vi "RW Limits Array.vi"(0 "Refnum In":T1, 2 "Read (F)":bool, 7 "LimitsArray In":cluster{"Step":dbl, "Max":dbl, "Min":dbl}[](array[cluster]), 11 "Error In":errorcluster) -> (4 "Refnum Out":T1, 8 "LimitsArray Out":cluster{"Step":dbl, "Max":dbl, "Min":dbl}[](array[cluster]), 15 "Error Out":errorcluster)   [LabVIEW 2013]
uses:
  <vilib>/Utility/config.llb/Config Data RefNum.ctl
  <vilib>/Utility/config.llb/Write Key (Double).vi
  <vilib>/Utility/config.llb/Read Key (Double).vi
  <vilib>/Utility/config.llb/NI_LVConfig.lvlib
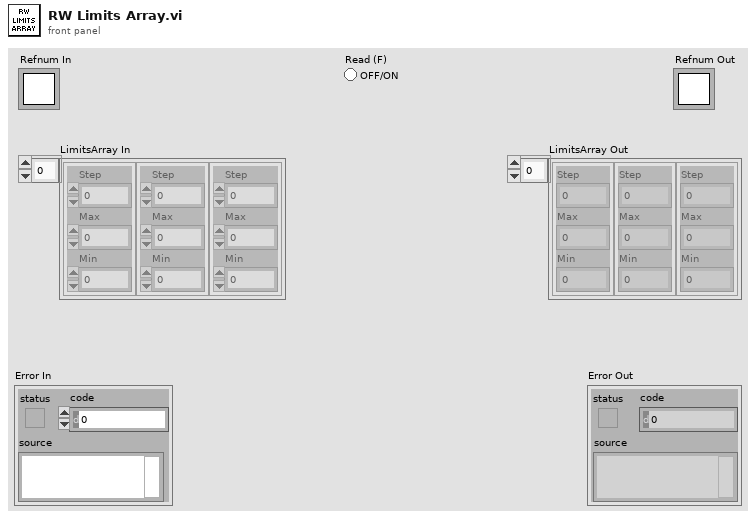
[diagram p1: front panel]
types:
  T1 = typedef "NI_LVConfig.lvlib/Config Data RefNum.ctl" = refnum<k1>
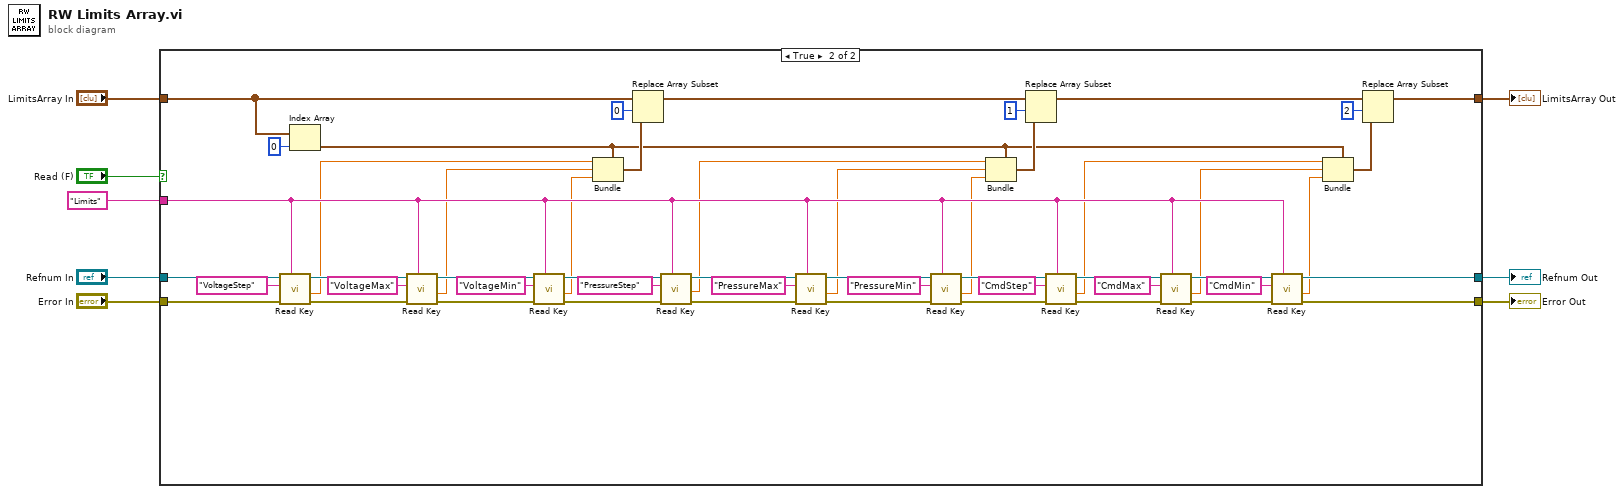
[diagram p0: block diagram]
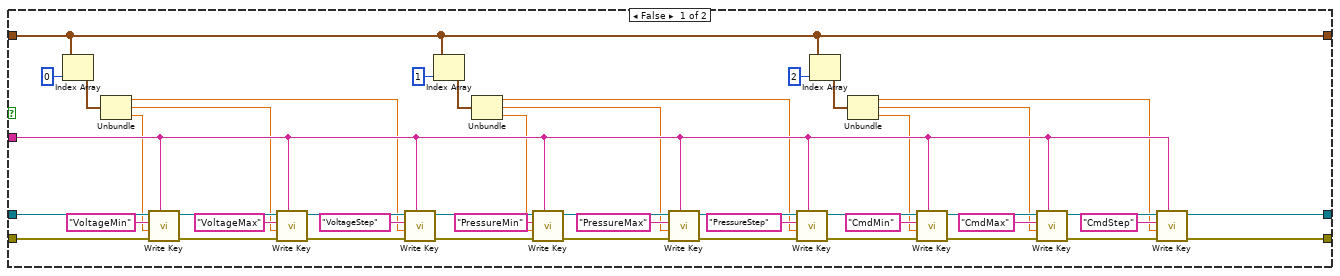
[diagram p2: hidden frame]
diagram:
  n1 = case shown="True" "Read (F)" {
    tunnel: "Error In" -> [w54 w104]
    tunnel: [w45 w94] -> w7
    tunnel: "Refnum In" -> [w44 w105]
    tunnel: [w35 w95] -> w4
    tunnel: "Limits" ("section") -> [w34 w85]
    tunnel: "LimitsArray In" -> [w27 w74]
    tunnel: [w27 w71] -> w1
    frame False {
      n2 = Index Array(array=w27, index=0) -> (element=w33:cluster{"Step":dbl, "Max":dbl, "Min":dbl})
      n3 = Unbundle(w33) -> ("Step"=w15:dbl, "Max"=w16:dbl, "Min"=w17:dbl)
      n4 = call-poly <vilib>:"Write Key.vi"("section"=w34, "error in (no error)"=w54, "value"=w17, "key"="VoltageMin", "refnum"=w44) -> ("error out"=w53:errorcluster, "refnum out"=w43:T1)  [unwired: 4 in, 1 out]
      n5 = call-poly <vilib>:"Write Key.vi"("section"=w34, "error in (no error)"=w53, "value"=w16, "key"="VoltageMax", "refnum"=w43) -> ("error out"=w52:errorcluster, "refnum out"=w42:T1)  [unwired: 4 in, 1 out]
      n6 = call-poly <vilib>:"Write Key.vi"("section"=w34, "error in (no error)"=w52, "value"=w15, "key"="VoltageStep", "refnum"=w42) -> ("error out"=w51:errorcluster, "refnum out"=w41:T1)  [unwired: 4 in, 1 out]
      n7 = Index Array(array=w27, index=1) -> (element=w30:cluster{"Step":dbl, "Max":dbl, "Min":dbl})
      n8 = Unbundle(w30) -> ("Step"=w12:dbl, "Max"=w13:dbl, "Min"=w14:dbl)
      n9 = call-poly <vilib>:"Write Key.vi"("section"=w34, "error in (no error)"=w51, "value"=w14, "key"="PressureMin", "refnum"=w41) -> ("error out"=w50:errorcluster, "refnum out"=w40:T1)  [unwired: 4 in, 1 out]
      n10 = call-poly <vilib>:"Write Key.vi"("section"=w34, "error in (no error)"=w50, "value"=w13, "key"="PressureMax", "refnum"=w40) -> ("error out"=w49:errorcluster, "refnum out"=w39:T1)  [unwired: 4 in, 1 out]
      n11 = call-poly <vilib>:"Write Key.vi"("section"=w34, "error in (no error)"=w49, "value"=w12, "key"="PressureStep", "refnum"=w39) -> ("error out"=w48:errorcluster, "refnum out"=w38:T1)  [unwired: 4 in, 1 out]
      n12 = Index Array(array=w27, index=2) -> (element=w29:cluster{"Step":dbl, "Max":dbl, "Min":dbl})
      n13 = Unbundle(w29) -> ("Step"=w9:dbl, "Max"=w10:dbl, "Min"=w11:dbl)
      n14 = call-poly <vilib>:"Write Key.vi"("section"=w34, "error in (no error)"=w48, "value"=w11, "key"="CmdMin", "refnum"=w38) -> ("error out"=w47:errorcluster, "refnum out"=w37:T1)  [unwired: 4 in, 1 out]
      n15 = call-poly <vilib>:"Write Key.vi"("section"=w34, "error in (no error)"=w47, "value"=w10, "key"="CmdMax", "refnum"=w37) -> ("error out"=w46:errorcluster, "refnum out"=w36:T1)  [unwired: 4 in, 1 out]
      n16 = call-poly <vilib>:"Write Key.vi"("section"=w34, "error in (no error)"=w46, "value"=w9, "key"="CmdStep", "refnum"=w36) -> ("error out"=w45:errorcluster, "refnum out"=w35:T1)  [unwired: 4 in, 1 out]
    }
    frame True {
      n17 = call-poly <vilib>:"Read Key.vi"("section"=w85, "error in (no error)"=w104, "key"="VoltageStep", "refnum"=w105) -> ("error out"=w86:errorcluster, "value"=w55:dbl, "refnum out"=w103:T1)  [unwired: 4 in, 1 out]
      n18 = Index Array(array=w74, index=0) -> (element=w68:cluster{"Step":dbl, "Max":dbl, "Min":dbl})
      n19 = call-poly <vilib>:"Read Key.vi"("section"=w85, "error in (no error)"=w86, "key"="VoltageMax", "refnum"=w103) -> ("error out"=w87:errorcluster, "value"=w56:dbl, "refnum out"=w102:T1)  [unwired: 4 in, 1 out]
      n20 = call-poly <vilib>:"Read Key.vi"("section"=w85, "error in (no error)"=w87, "key"="VoltageMin", "refnum"=w102) -> ("error out"=w88:errorcluster, "value"=w57:dbl, "refnum out"=w101:T1)  [unwired: 4 in, 1 out]
      n21 = Bundle(cluster=w68, "Step"=w55, "Max"=w56, "Min"=w57) -> (w70:cluster{"Step":dbl, "Max":dbl, "Min":dbl})
      n22 = Replace Array Subset(array=w74, new element=w70, index=0) -> (w73:cluster{"Step":dbl, "Max":dbl, "Min":dbl}[])
      n23 = call-poly <vilib>:"Read Key.vi"("section"=w85, "error in (no error)"=w88, "key"="PressureStep", "refnum"=w101) -> ("error out"=w89:errorcluster, "value"=w58:dbl, "refnum out"=w100:T1)  [unwired: 4 in, 1 out]
      n24 = call-poly <vilib>:"Read Key.vi"("section"=w85, "error in (no error)"=w89, "key"="PressureMax", "refnum"=w100) -> ("error out"=w90:errorcluster, "value"=w59:dbl, "refnum out"=w99:T1)  [unwired: 4 in, 1 out]
      n25 = call-poly <vilib>:"Read Key.vi"("section"=w85, "error in (no error)"=w90, "key"="PressureMin", "refnum"=w99) -> ("error out"=w91:errorcluster, "value"=w60:dbl, "refnum out"=w98:T1)  [unwired: 4 in, 1 out]
      n26 = Bundle(cluster=w68, "Step"=w58, "Max"=w59, "Min"=w60) -> (w69:cluster{"Step":dbl, "Max":dbl, "Min":dbl})
      n27 = Replace Array Subset(array=w73, new element=w69, index=1) -> (w72:cluster{"Step":dbl, "Max":dbl, "Min":dbl}[])
      n28 = call-poly <vilib>:"Read Key.vi"("section"=w85, "error in (no error)"=w91, "key"="CmdStep", "refnum"=w98) -> ("error out"=w92:errorcluster, "value"=w61:dbl, "refnum out"=w97:T1)  [unwired: 4 in, 1 out]
      n29 = call-poly <vilib>:"Read Key.vi"("section"=w85, "error in (no error)"=w92, "key"="CmdMax", "refnum"=w97) -> ("error out"=w93:errorcluster, "value"=w62:dbl, "refnum out"=w96:T1)  [unwired: 4 in, 1 out]
      n30 = call-poly <vilib>:"Read Key.vi"("section"=w85, "error in (no error)"=w93, "key"="CmdMin", "refnum"=w96) -> ("error out"=w94:errorcluster, "value"=w63:dbl, "refnum out"=w95:T1)  [unwired: 4 in, 1 out]
      n31 = Bundle(cluster=w68, "Step"=w61, "Max"=w62, "Min"=w63) -> (w67:cluster{"Step":dbl, "Max":dbl, "Min":dbl})
      n32 = Replace Array Subset(array=w72, new element=w67, index=2) -> (w71:cluster{"Step":dbl, "Max":dbl, "Min":dbl}[])
    }
  }
  "Refnum Out" <- w4
  "Error Out" <- w7
  "LimitsArray Out" <- w1
